vi "Read Type.vi"(8 "error in (no error)":errorcluster, 11 "ODESimulator_Base_Conveyor in":refnum<class "ODESimulator_Base_Conveyor.lvclass">) -> (0 "error out":errorcluster, 2 "Type":string, 3 "ODESimulator_Base_Conveyor out":refnum<class "ODESimulator_Base_Conveyor.lvclass">)   [LabVIEW 2017, in "NI_Robotics_Simulator.lvlib" / "ODESimulator_Base_Conveyor.lvclass"]
uses:
  <vilib>/robotics/Simulator/Robot Factory/Conveyor/Base/ODESimulator_Base_Conveyor.lvclass
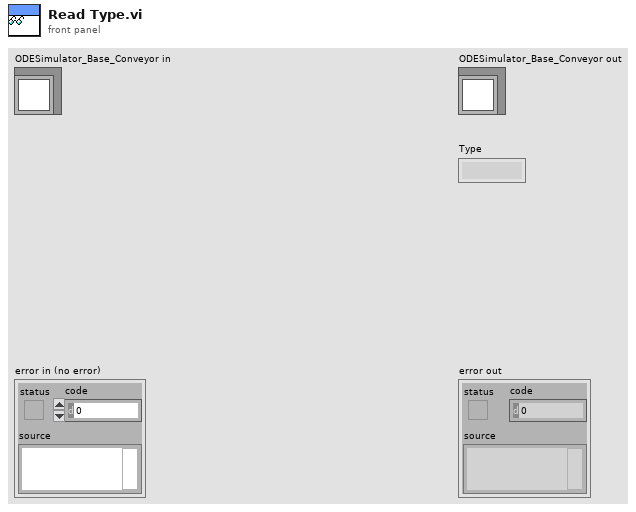
[diagram p1: front panel]
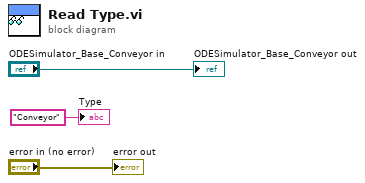
[diagram p0: block diagram]
diagram:
  "error out" <- "error in (no error)"
  "ODESimulator_Base_Conveyor out" <- "ODESimulator_Base_Conveyor in"
  "Type" <- "Conveyor" ("Type")
